vi "labview-system-logging-example.vi"() -> ()   [LabVIEW 2021]
uses:
  source/system.logging/system.logging.lvclass
panel:
  out "exit_code":i32
  in  "stop":bool
  in  "configuration path":path
  # "This VI provides and example of the system.logging tool.\n\nINSTRUCTIONS:\n1. Specify the path to logging.config, this is the JSON configuration file that specifies logging providers.\n2. Review the provider configuration.\n3. Run the VI.\n\nCTRL+E to view block diagram."
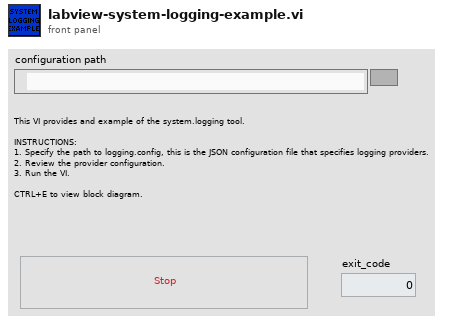
[diagram p1: front panel]
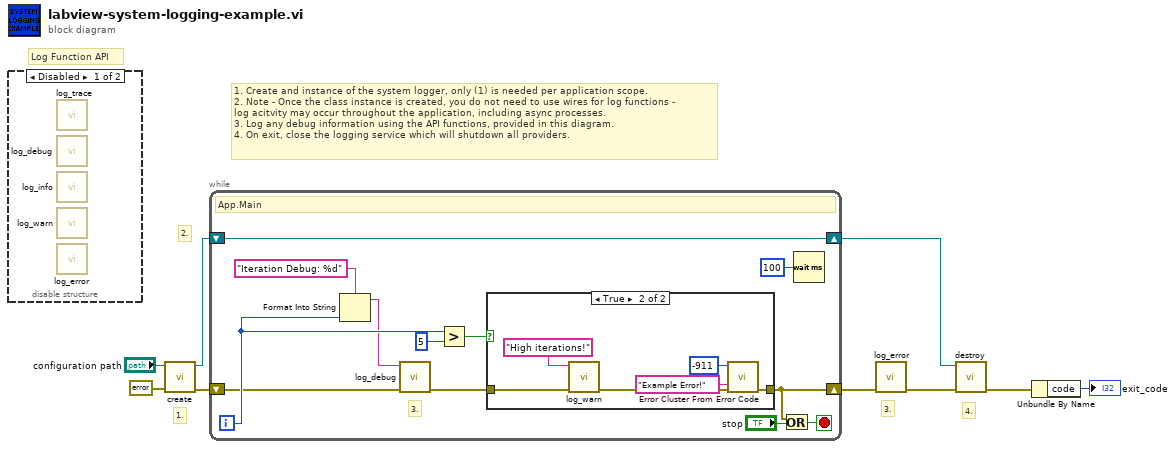
[diagram p0: block diagram]
diagram:
  # "Log Function API"
  # "4."
  # "3."
  # "2."
  # "1."
  # "1. Create and instance of the system logger, only (1) is needed per application scope.\n2. Note - Once the class instance is created, you do not need to use wires for log functions -\nlog acitvity may occur throughout the application, including async processes.\n3. Log any debug information using the API functions, provided in this diagram.\n4. On exit, close the logging service which will shutdown all providers."
  n1 = disable-structure shown="Disabled" {
    frame Disabled {
      n2 = call "log_trace.vi"() -> ()  [unwired: 11 in, 1 out]
      n3 = call "log_debug.vi"() -> ()  [unwired: 11 in, 1 out]
      n4 = call "log_info.vi"() -> ()  [unwired: 11 in, 1 out]
      n5 = call "log_warn.vi"() -> ()  [unwired: 11 in, 1 out]
      n6 = call "log_error.vi"() -> ()  [unwired: 11 in, 1 out]
    }
    frame Enabled {
    }
  }
  n7 = call "create.vi"("error in (no error)"=errorcluster {"status"=FALSE, "code"=0, "source"=""}, "path"="configuration path") -> ("error out"=w6:errorcluster, "logging"=w7:refnum<class "system.logging.lvclass">)  [unwired: 8 in]
  n8 = while {
    shift-right: [w21] -> w1
    shift-left: w7 -> [w21]
    shift-right: [w14] -> w5
    shift-left: w6 -> [w12]
    i -> [w17]
    stop <- w20 stop-if-true
    # "3."
    # "App.Main"
    n9 = Format Into String(format string="Iteration Debug: %d", w17) -> (resulting string=w10:string)  [unwired: 2 in, 1 out]
    n10 = call "log_debug.vi"("error in (no error)"=w12, "message"=w10) -> ("error out"=w11:errorcluster)  [unwired: 9 in]
    n11 = Greater?(x=w17, y=5) -> (0:w15:bool)
    n12 = case shown="True" w15 {
      tunnel: w11 -> [w22 w28]
      tunnel: [w22 w25] -> w14
      frame False {
      }
      frame True {
        n13 = call "log_warn.vi"("error in (no error)"=w28, "message"="High iterations!") -> ("error out"=w26:errorcluster)  [unwired: 9 in]
        n14 = call <vilib>:"Error Cluster From Error Code.vi"("error in (no error)"=w26, "error message (\"\")"="Example Error!" ("error message (\"\")"), "error code (0)"=-911) -> ("error out"=w25:errorcluster)  [unwired: 6 in]
      }
    }
    n15 = Or(x=w14, y="stop") -> (x .or. y?=w20:bool)
    n16 = Wait (ms)(milliseconds to wait=u32 100) -> ()  [unwired: 1 out]
  }
  n17 = call "log_error.vi"("error in (no error)"=w5) -> ("error out"=w3:errorcluster)  [unwired: 10 in]
  n18 = call "destroy.vi"("error in (no error)"=w3, "system.logging in"=w1) -> ("error out"=w2:errorcluster)  [unwired: 9 in]
  n19 = Unbundle By Name(w2) -> ("code"=→"exit_code":i32)
